vi "Update XY Plots.vi"(8 "error in (no error)":errorcluster, 9 "Persistent Data.Graph Props.Legend:Number of Rows":u32, 10 "Plots":T1[](array[typedef]), 11 "Graph":refnum<vi>) -> (0 "error out":errorcluster)   [LabVIEW 2020, in "Workspace MultiY Graph.lvlib"]
uses:
  Workspace MultiY Graph.lvlib
  XY Plot Properties.ctl
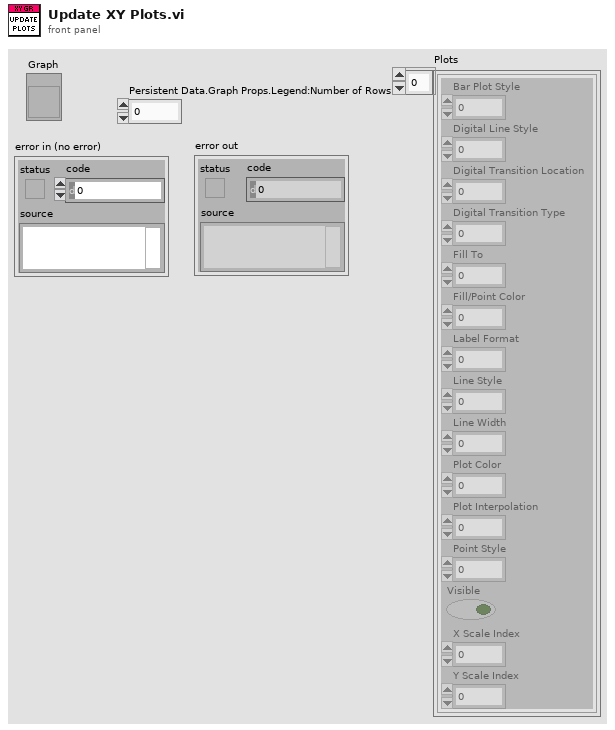
[diagram p1: front panel]
types:
  T1 = typedef "Workspace MultiY Graph.lvlib/XY Plot Properties.ctl" = cluster{"Bar Plot Style":u8, "Digital Line Style":u8, "Digital Transition Location":u8, "Digital Transition Type":u8, "Fill To":i16, "Fill/Point Color":u32, "Label Format":u8, "Line Style":u8, "Line Width":u8, "Plot Color":u32, "Plot Interpolation":u8, "Point Style":u8, "Visible":bool, "X Scale Index":u32, "Y Scale Index":u32}
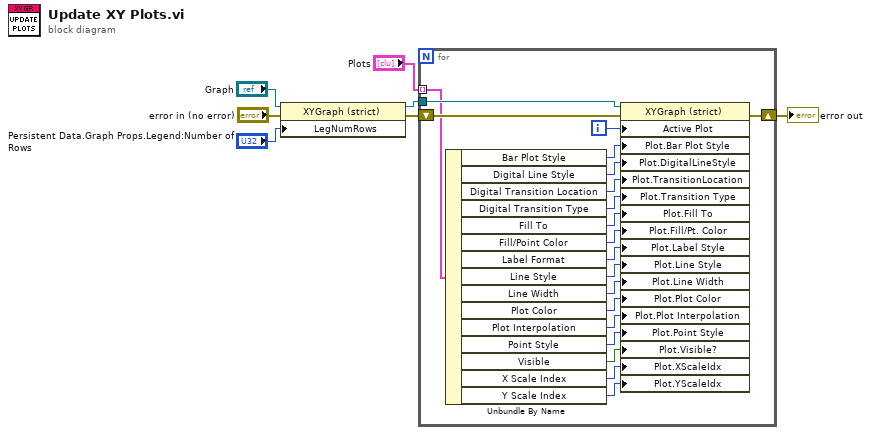
[diagram p0: block diagram]
diagram:
  n1 = property class="XYGraph (strict)"(reference="Graph", error in="error in (no error)", "LegNumRows"="Persistent Data.Graph Props.Legend:Number of Rows") -> (reference out=w3:refnum<vi>, error out=w4:errorcluster)
  n2 = for {
    tunnel: "Plots" -> [w23] mode=indexing
    shift-right: [w24] -> w6
    shift-left: w4 -> [w27]
    tunnel: w3 -> [w26]
    i -> [w25]
    n3 = Unbundle By Name(w23) -> ("Bar Plot Style"=w22:u8, "Digital Line Style"=w21:u8, "Digital Transition Location"=w20:u8, "Digital Transition Type"=w19:u8, "Fill To"=w18:i16, "Fill/Point Color"=w17:u32, "Label Format"=w16:u8, "Line Style"=w15:u8, "Line Width"=w14:u8, "Plot Color"=w13:u32, "Plot Interpolation"=w12:u8, "Point Style"=w11:u8, "Visible"=w10:bool, "X Scale Index"=w9:u32, "Y Scale Index"=w8:u32)
    n4 = property class="XYGraph (strict)"(reference=w26, error in=w27, "Active Plot"=w25, "Plot.Bar Plot Style"=w22, "Plot.DigitalLineStyle"=w21, "Plot.TransitionLocation"=w20, "Plot.Transition Type"=w19, "Plot.Fill To"=w18, "Plot.Fill/Pt. Color"=w17, "Plot.Label Style"=w16, "Plot.Line Style"=w15, "Plot.Line Width"=w14, "Plot.Plot Color"=w13, "Plot.Plot Interpolation"=w12, "Plot.Point Style"=w11, "Plot.Visible?"=w10, "Plot.XScaleIdx"=w9, "Plot.YScaleIdx"=w8) -> (error out=w24:errorcluster)  [unwired: 1 out]
  }
  "error out" <- w6
